vi "hReadChannelsRTDMA2013.vi"(0 "FPGA VI Reference In":refnum<k20>, 1 "Nsamples":u32, 3 "error in":errorcluster) -> (5 "FPGA VI Reference Out":refnum<k20>, 6 "Fehler":bool, 7 "RawArray":i16[][](array[numeric]), 8 "error out":errorcluster)   [LabVIEW 2014]
doc: "startet das einlesen und führt dies bis n Samples aus\nHier mit FIFO und IRQ."
uses:
  <vilib>/Utility/error.llb/Error Cluster From Error Code.vi
  <vilib>/rvi/errors/niLvFpgaAdjustHostInterfaceError.vi
  <vilib>/RVI Host/nirviSupport.llb/nirviErrorClusterFromErrorCode.vi
  <vilib>/rvi/interface/nirviReadWriteControl/nirviReadWriteControl.xnode
  FPGA Bitfiles/W7XBolo2017_FPGATarget_fmain2014_9xlV3GyHFfo.lvbitx
  f_main_2014.vi
  <vilib>/rvi/interface/nirviMethod/nirviMethod.xnode
  NiFpgaLv.dll
  <vilib>/rvi/interface/nirviMethod/StockFPGA_InlinedMethodWaitForSingleIRQ.vi
  <vilib>/FPGAPlugInAG/PCI-7813R/niLvFpga_WaitOnIrq_PCI-7813R.vi
  <vilib>/FPGAPlugInAG/PCI-7813R/niLvFpga_AcknowledgeIrq_PCI-7813R.vi
  <vilib>/FPGAPlugInAG/PCI-7813R/niLvFpga_ReadFifo_PCI-7813R.vi
  <vilib>/rvi/errors/niLvFpgaMergeErrorWithErrorCode.vi
panel:
  out "error out source":string
  out "error out code":i32
  out "error out status":bool
  out "error out 4":errorcluster
  out "error out 3":errorcluster
  out "error out 2":errorcluster
  out "Fifo-Fehler":bool
  out "scanID > NSamples":bool
  out "rt fifo read element out":bool
  out "STOP?":bool
  out "ScanID":u32
  out "IRQ(s) Asserted":i32
  out "Timed Out":bool
  # "Sampling"
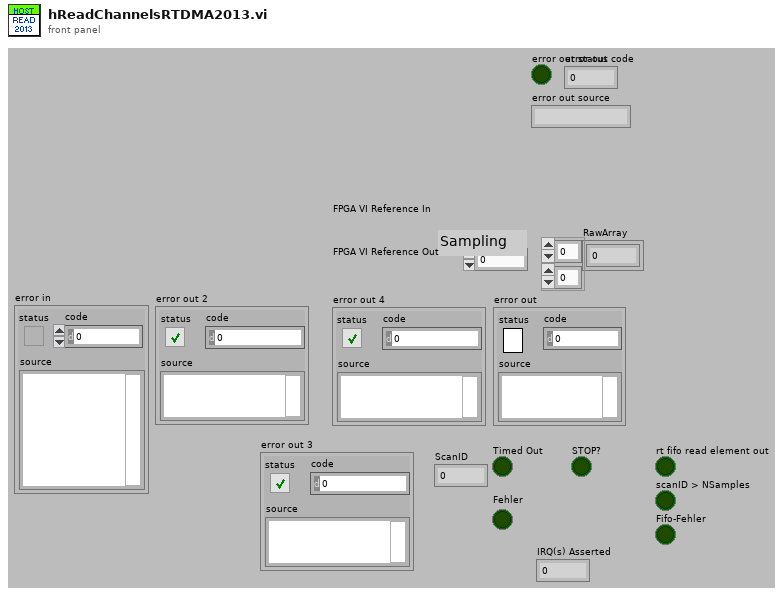
[diagram p1: front panel]
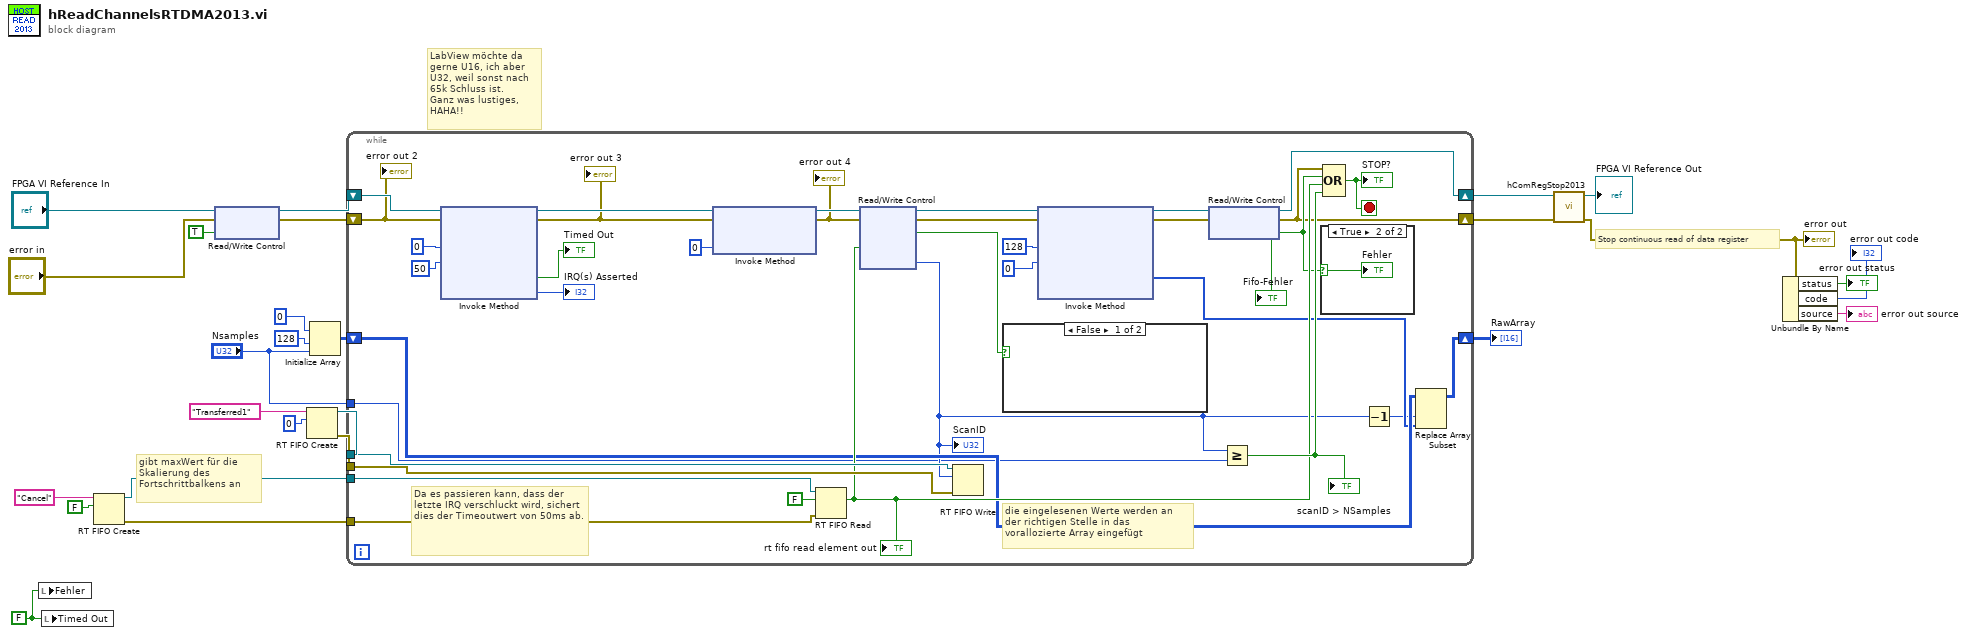
[diagram p0: block diagram]
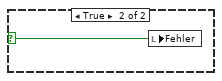
[diagram p3: hidden frame]
diagram:
  w18 = FALSE
  # "Stop continuous read of data register"
  # "gibt maxWert für die Skalierung des Fortschrittbalkens an"
  # "LabView möchte da gerne U16, ich aber U32, weil sonst nach 65k Schluss ist. \nGanz was lustiges, HAHA!!"
  n1 = local write "Fehler"(w18) -> ()
  n2 = local write "Timed Out"(w18) -> ()
  n3 = RT FIFO Create(0:"Cancel" ("name (unnamed)"), 1:FALSE) -> (8:w20:refnum<k33>, 11:w19:errorcluster)  [unwired: 2 in, 5 out]
  n4 = xnode "Read/Write Control"("FPGA VI Reference In"="FPGA VI Reference In", "error in"="error in", "ADCRead"=TRUE) -> ("FPGA VI Reference Out"=w11:refnum<k20>, "error out"=w10:errorcluster)
  n5 = RT FIFO Create(0:"Transferred1" ("name (unnamed)"), 1:u32 0) -> (8:w23:refnum<k33>, 11:w22:errorcluster)  [unwired: 2 in, 5 out]
  n6 = Initialize Array(i16 0, 128 ("dimension size"), "Nsamples") -> (w26:i16[][])
  n7 = while {
    tunnel: "Nsamples" -> [w28]
    shift-right: [w51] -> w15
    shift-left: w26 -> [w38]
    shift-right: [w58] -> w8
    shift-left: w11 -> [w60]
    shift-right: [w29] -> w9
    shift-left: w10 -> [w27]
    tunnel: w23 -> [w49]
    tunnel: w22 -> [w48]
    tunnel: w20 -> [w46]
    tunnel: w19 -> [w45]
    stop <- w50 stop-if-true
    # "die eingelesenen Werte werden an der richtigen Stelle in das vorallozierte Array eingefügt"
    # "Da es passieren kann, dass der letzte IRQ verschluckt wird, sichert dies der Timeoutwert von 50ms ab."
    n8 = xnode "Invoke Method"("FPGA VI Reference In"=w60, "error in"=w27, "IRQ Number(s)"=0, "Timeout (ms)"=50) -> ("FPGA VI Reference Out"=w57:refnum<k20>, "error out"=w56:errorcluster, "Timed Out"=→"Timed Out":bool, "IRQ(s) Asserted"=→"IRQ(s) Asserted":i32)
    "error out 3" <- w56
    n9 = xnode "Invoke Method"("FPGA VI Reference In"=w57, "error in"=w56, "IRQ Number(s)"=0 ("IRQ Number")) -> ("FPGA VI Reference Out"=w54:refnum<k20>, "error out"=w53:errorcluster)
    "error out 4" <- w53
    n10 = RT FIFO Read(0:w46, 1:FALSE ("element"), 3:w45) -> (9:w47:bool)  [unwired: 5 out]
    "rt fifo read element out" <- w47
    n11 = xnode "Read/Write Control"("FPGA VI Reference In"=w54, "error in"=w53, "cancel"=w47) -> ("FPGA VI Reference Out"=w40:refnum<k20>, "error out"=w39:errorcluster, "Timeout"=w43:bool, "ScanID"=w34:u32)
    "ScanID" <- w34
    n12 = RT FIFO Write(0:w49, 1:w34, 3:w48) -> ()  [unwired: 1 in, 5 out]
    n13 = case shown="False" w43 {
      selector: w43 -> [_ w63]
      frame False {
      }
      frame True {
        n14 = local write "Fehler"(w63) -> ()
      }
    }
    n15 = xnode ("Invoke Method")("FPGA VI Reference In"=w40, "error in"=w39, "Number of Elements"=u32 128, "Timeout (ms)"=0 ("Timeout")) -> ("FPGA VI Reference Out"=w32:refnum<k20>, "error out"=w31:errorcluster, "Data"=w37:u32[])  [unwired: 1 out]
    n16 = xnode "Read/Write Control"("FPGA VI Reference In"=w32, "error in"=w31) -> ("FPGA VI Reference Out"=w58:refnum<k20>, "error out"=w29:errorcluster, "Fifo-Fehler"=w30:bool)
    "Fifo-Fehler" <- w30
    n17 = Greater Or Equal?(x=w34, y=w28) -> (x >= y?=w61:bool)
    "scanID > NSamples" <- w61
    n18 = case shown="True" w30 {
      selector: w30 -> [_ w62]
      frame False {
      }
      frame True {
        "Fehler" <- w62
      }
    }
    n19 = Compound Arithmetic op=OR(w29, w30, w47, w61) -> (w50:bool)
    "STOP?" <- w50
    n20 = Decrement(x=w34) -> (x-1=w33:u32)
    n21 = Replace Array Subset(array=w38, new element=w37, index (col)=w33) -> (w51:i16[][])  [unwired: 1 in]
    "error out 2" <- w27
  }
  "RawArray" <- w15
  n22 = call "hComRegStop2013.vi"("error in"=w9, "FPGA VI Reference In"=w8) -> ("error out"=w4:errorcluster, "FPGA VI Reference Out"=→"FPGA VI Reference Out":refnum<k20>)  [unwired: 3 in, 1 out]
  "error out" <- w4
  n23 = Unbundle By Name(w4) -> ("status"=→"error out status":bool, "code"=→"error out code":i32, "source"=→"error out source":string)
